vi "Pre Launch Init.vi"(11 "Nested in":refnum<class "UI Template with RefNums FBCtrl.lvclass">) -> (0 "error out":errorcluster, 3 "Nested out":refnum<class "UI Template with RefNums FBCtrl.lvclass">)   [LabVIEW 2020, in "UI Template with RefNums FBCtrl.lvclass"]
doc: "(<B>Filename</B>: Actor Framework.lvlib:Actor.lvclass:Pre Launch Init.vi)\n\nDefines behavior that occurs after the Launch Nested Actor method is invoked but before the actor's Actor Core method begins running.\n\nBy default, this method does nothing. A descendant class may override it to define behavior."
uses:
  UI Template with RefNums FBCtrl.lvclass
  UI Template with RefNums FBCtrl.lvclass/UI Template with RefNums FBCtrl.ctl
  <vilib>/ActorFramework/Actor/Actor.lvclass
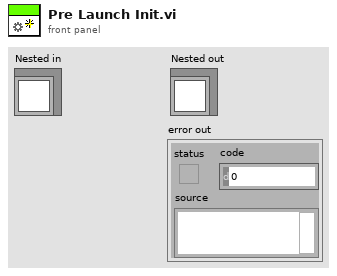
[diagram p1: front panel]
types:
  T1 = enum32{"Invalid", "Standard", "Closed", "Hidden", "Minimized", "Maximized"}
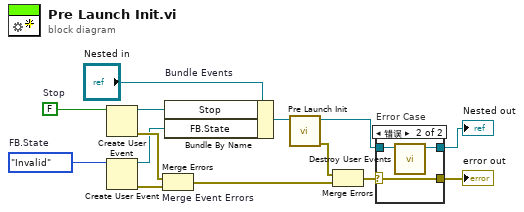
[diagram p0: block diagram]
diagram:
  w3 = T1."Invalid"  # FB.State
  w13 = FALSE  # Stop
  n1 = Create User Event(user event datatype=w13) -> (user event=w10:refnum<user-event>, error out=w12:errorcluster)  [unwired: 1 in]
  n2 = Create User Event(user event datatype=w3) -> (user event=w2:refnum<user-event>, error out=w1:errorcluster)  [unwired: 1 in]
  n3 = Merge Errors "Merge Event Errors"(w12, w1) -> (w4:errorcluster)
  n4 = Bundle By Name "Bundle Events"(cluster="Nested in", "Stop"=w10, "FB.State"=w2) -> (w7:refnum<class "UI Template with RefNums FBCtrl.lvclass">)
  n5 = call-parent "Pre Launch Init.vi"("Actor in"=w7) -> ("error out"=w6:errorcluster, "Actor out"=w8:refnum<class "UI Template with RefNums FBCtrl.lvclass">)  [unwired: 9 in]
  n6 = Merge Errors ("合并错误")(w6, w4) -> (w5:errorcluster)
  n7 = case "Error Case" shown="错误" w5 {
    selector: w5 -> [w15 w19]
    tunnel: w8 -> [w16 w18]
    tunnel: [w16 w17] -> w11
    tunnel: [w15 w19] -> w9
    frame No Error {
    }
    frame Error {
      n8 = call "Destroy User Events.vi"("UI Template in"=w18) -> ("UI Template out"=w17:refnum<class "UI Template with RefNums FBCtrl.lvclass">)  [unwired: 10 in]
    }
  }
  "error out" <- w9
  "Nested out" <- w11
